vi "Main.vi"() -> ()   [LabVIEW 2020, in "Main.lvclass"]
uses:
  Main/Main.lvclass
  Support/Log Indicator/Log Indicator.lvclass
  C:/Program Files (x86)/National Instruments/LabVIEW 2020/vi.lib/Asteme/Triarc Framework/Logging/Logging.lvclass
  Main/Main.lvclass/Main.ctl
  Support/Log Indicator/Log Indicator.lvclass/Log Indicator.ctl
  <vilib>/Asteme/Triarc Framework/Process/Process.lvclass/Process.ctl
  <vilib>/Asteme/Triarc Framework/Process/Private/SubVIs/Wait for finish.vi
  <vilib>/Asteme/Triarc Framework/Process/Protected/Messaging/Enqueue Message.vi
  <vilib>/Asteme/Triarc Framework/Process/Private/SubVIs/Set Lifecycle State.vi
  <vilib>/Asteme/Triarc Framework/Process/Public/Lifecycle/Get Lifecycle State.vi
  <vilib>/Utility/error.llb/Clear Errors.vi
  Processes/Coffee Shop/Coffee Shop.lvclass
  C:/Program Files (x86)/National Instruments/LabVIEW 2020/vi.lib/Asteme/Triarc Framework/Process/Process.lvclass
  C:/Program Files (x86)/National Instruments/LabVIEW 2020/vi.lib/Asteme/Triarc Framework/Application/Application.lvclass
  <vilib>/Utility/error.llb/Error Cluster From Error Code.vi
  <vilib>/Asteme/Triarc Framework/Application/Application.lvclass
  <vilib>/Asteme/Triarc Framework/Process/Process.lvclass
panel:
  in  "Has Phone?":bool=TRUE
  out "System Log":string
  in  "Remove Customer":bool
  in  "Stop Button":bool
  in  "Remove Barista":bool
  in  "Show Barista Info":bool
  in  "Add Barista":bool
  in  "Baristas":i32(listbox)=-1
  in  "Remove Cashier":bool
  in  "Show Cashier Info":bool
  in  "Add Cashier":bool
  in  "Cashiers":i32(listbox)=-1
  in  "Show Customer Info":bool
  in  "Add Customer":bool
  in  "Customers":i32(listbox)=-1
  # "Click + to add a customer actor to the system.\nClick Place Order to choose items for the customer to order.\nCustomer will wait until all items ordered are ready, then exit."
  # "Cashiers process orders into individual drink jobs and forwards those jobs to baristas.\nClick + to add a cashier actor to the system.\nClick - to remove a cashier from the system."
  # "Baristas process drink jobs and notify customers of completed drinks.\nAdd more baristas to the system by clicking +.  Pending jobs will be assigned to the next available barista.\nClick - to remove a barista from the system."
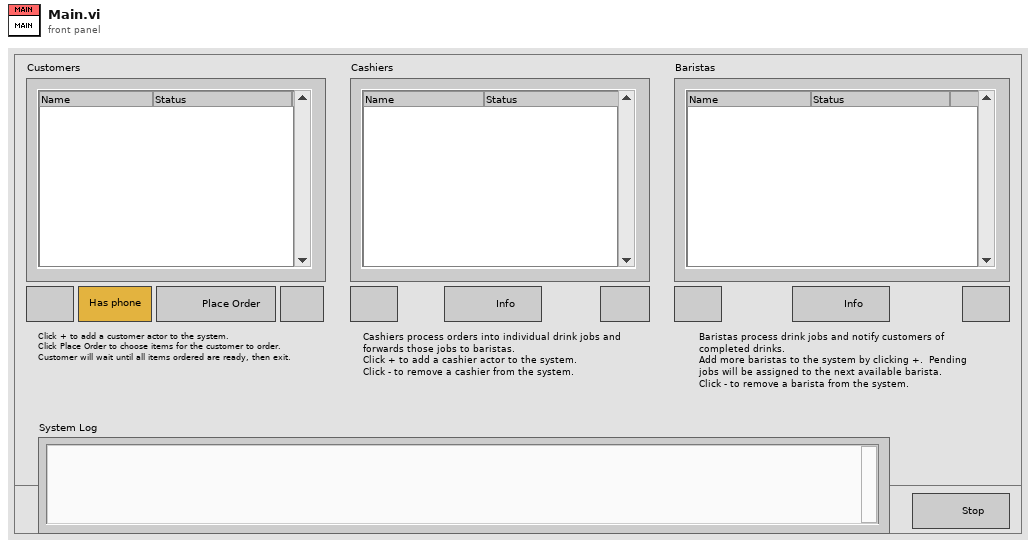
[diagram p1: front panel]
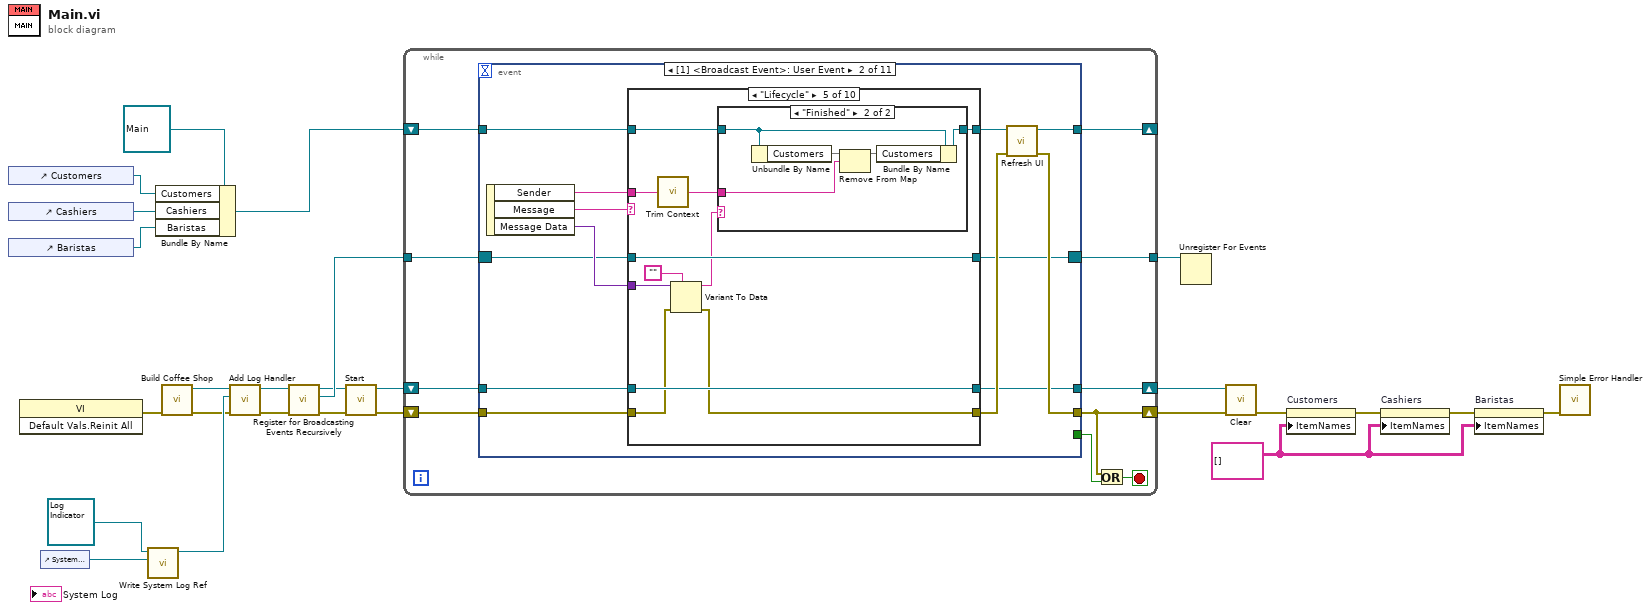
[diagram p0: block diagram]
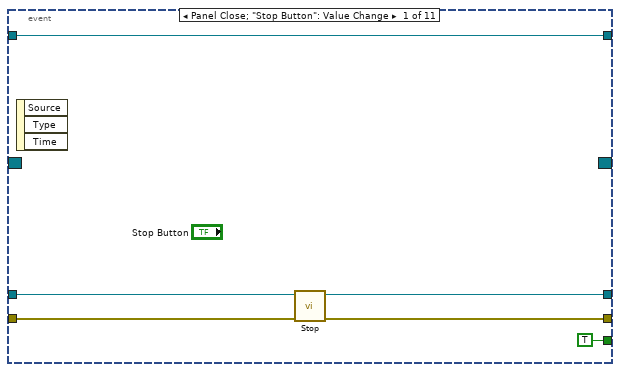
[diagram p2: hidden frame]
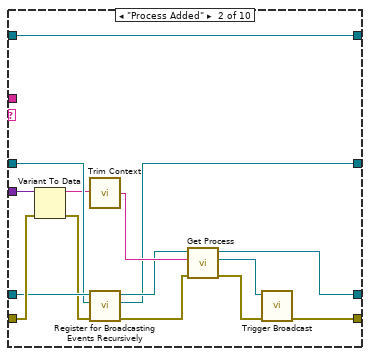
[diagram p4: hidden frame]
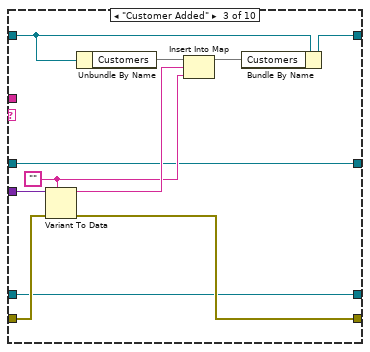
[diagram p5: hidden frame]
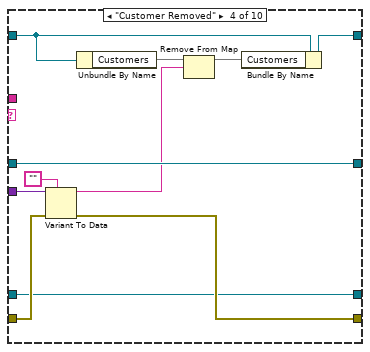
[diagram p6: hidden frame]
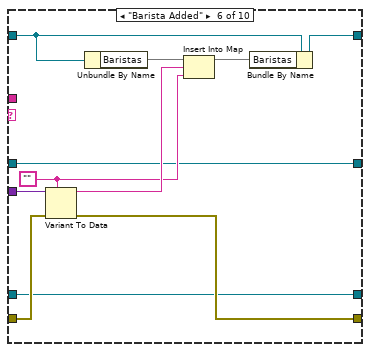
[diagram p8: hidden frame]
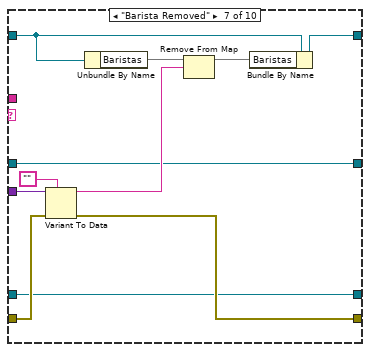
[diagram p9: hidden frame]
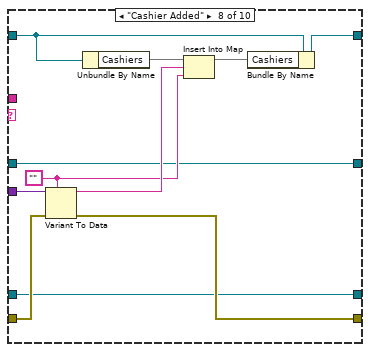
[diagram p10: hidden frame]
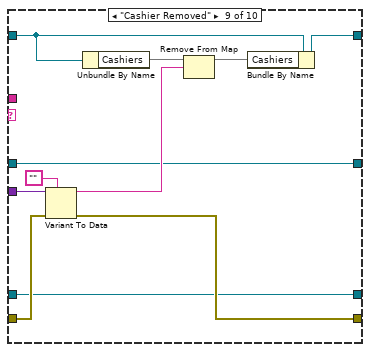
[diagram p11: hidden frame]
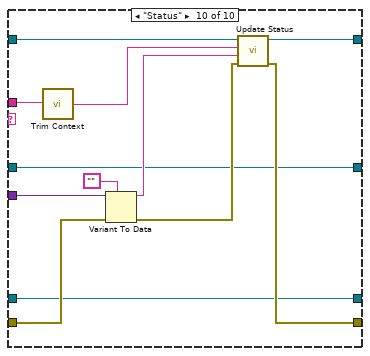
[diagram p12: hidden frame]
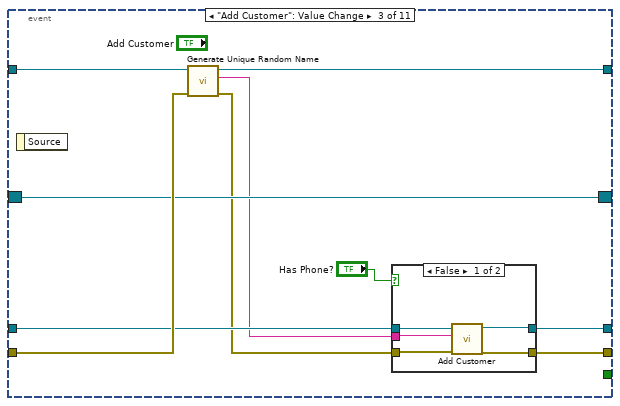
[diagram p13: hidden frame]
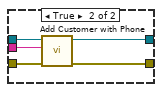
[diagram p14: hidden frame]
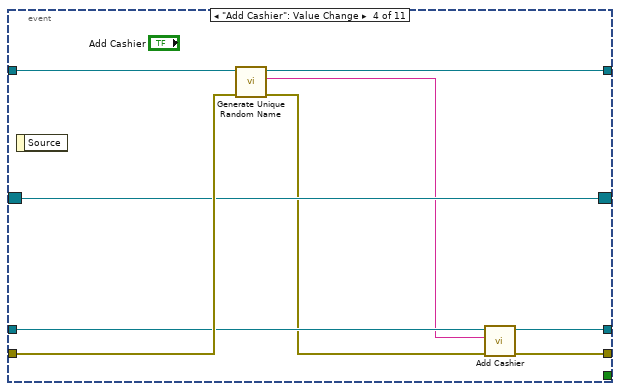
[diagram p15: hidden frame]
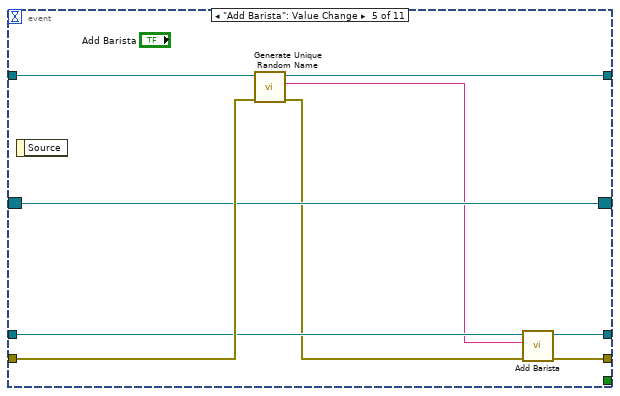
[diagram p16: hidden frame]
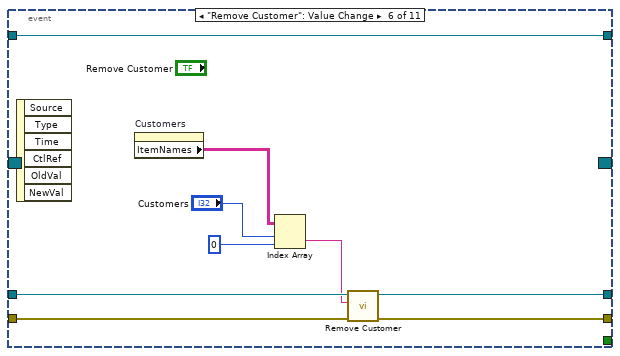
[diagram p17: hidden frame]
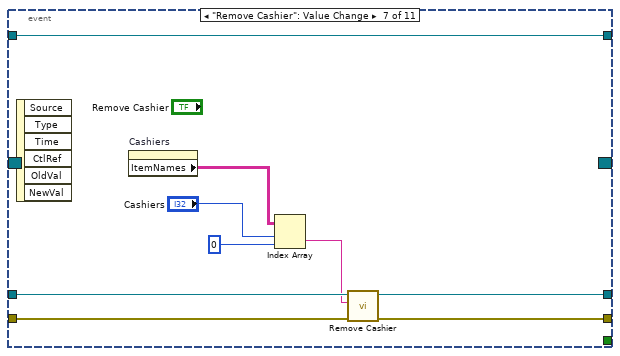
[diagram p18: hidden frame]
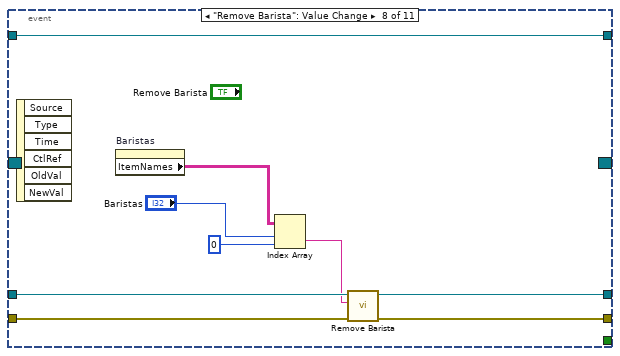
[diagram p19: hidden frame]
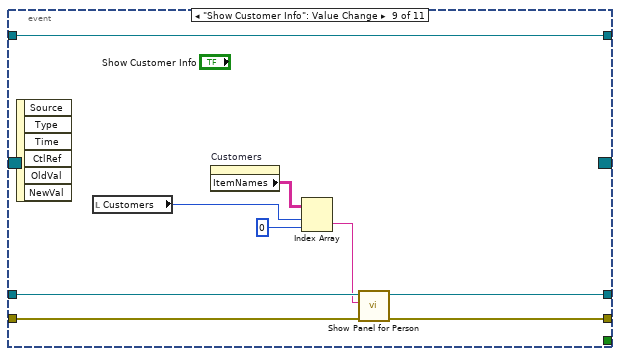
[diagram p20: hidden frame]
diagram:
  w8 = string[][] [] ("Item Names")
  n1 = control-ref of="Customers"() -> (w20:refnum<vi>)
  n2 = control-ref of="Cashiers"() -> (w19:refnum<vi>)
  n3 = control-ref of="Baristas"() -> (w18:refnum<vi>)
  n4 = invoke on="Invoke Node" class="VI" method="Default Vals.Reinit All"() -> (error out=w23:errorcluster)  [unwired: 3 in, 2 out]
  n5 = control-ref of="System Log"() -> (w14:refnum<vi>)
  n6 = call "Write System Log Ref.vi"("System Log"=w14, "Log Indicator in"=refnum<class "Log Indicator.lvclass"> refnum ("Log Indicator.lvclass")) -> ("Log Indicator out"=w12:refnum<class "Log Indicator.lvclass">)  [unwired: 8 in, 1 out]
  n7 = Bundle By Name(cluster=refnum<class "Main.lvclass"> refnum ("Main.lvclass"), "Customers"=w20, "Cashiers"=w19, "Baristas"=w18) -> (w21:refnum<class "Main.lvclass">)
  n8 = call "Build Coffee Shop.vi"("error in (no error)"=w23) -> ("error out"=w10:errorcluster, "Coffee Shop Out"=w11:refnum<class "Coffee Shop.lvclass">)  [unwired: 9 in]
  n9 = call <vilib>:"Add Log Handler.vi"("error in (no error)"=w10, "Log Handler"=w12, "Process In"=w11) -> ("error out"=w13:errorcluster, "Process Out"=w9:refnum<class "Coffee Shop.lvclass">)  [unwired: 7 in]
  n10 = call <vilib>:"Register for Broadcasting Events Recursively.vi"("error in (no error)"=w13, "Application In"=w9) -> ("error out"=w17:errorcluster, "Event Registration Refnum Out"=w16:refnum<event-registration>, "Application Out"=w3:refnum<class "Coffee Shop.lvclass">)  [unwired: 7 in]
  n11 = call <vilib>:"Start.vi"("error in (no error)"=w17, "Process In"=w3) -> ("error out"=w4:errorcluster, "Process Out"=w2:refnum<class "Coffee Shop.lvclass">)  [unwired: 8 in]
  n12 = while {
    shift-right: [w35] -> w25
    shift-left: w4 -> [w36]
    shift-right: [w31] -> w24
    shift-left: w2 -> [w32]
    tunnel: w16 -> [w30]
    tunnel: [w29] -> w26
    shift-right: [w27] -> _
    shift-left: w21 -> [w28]
    stop <- w34 stop-if-true
    n13 = event shown="[1] <Broadcast Event>: User Event" {
      selector: w30 -> [_ w44 w177 w196 w205 _ _ _ _ _ _]
      dyn-events: [_ w43 w177 w196 w205 _ _ _ _ _ _] -> w29
      timeout: _ -> [_ _ _ _ _ _ _ _ _ _ _]
      tunnel: [w40 w50 w175 w194 w203 w215 w224 w233 w238 w247 w256] -> w35
      tunnel: w36 -> [w42 w52 w179 w198 w207 w214 w223 w232 w243 w252 w261]
      tunnel: [TRUE _ _ _ _ _ _ _ _ _ _] -> w33
      tunnel: w32 -> [w39 w45 w178 w197 w206 w212 w221 w230 w237 w246 w255]
      tunnel: [w38 w46 w176 w195 w204 w213 w222 w231 w236 w245 w254] -> w31
      tunnel: w28 -> [w37 w51 w172 w192 w201 w216 w225 w234 w242 w251 w260]
      tunnel: [w37 w48 w171 w191 w200 w216 w225 w234 w242 w251 w260] -> w27
      event Panel Close; "Stop Button": Value Change {
        n14 = event-data() -> ()  [unwired: 1 in, 3 out]
        n15 = call <vilib>:"Stop.vi"("error in (no error)"=w42, "Process In"=w39) -> ("error out"=w40:errorcluster, "Process Out"=w38:refnum<class "Coffee Shop.lvclass">)  [unwired: 7 in, 1 out]
      }
      event User Event {
        n16 = event-data() -> ("Sender"=w47:string, "Message"=w55:string, "Message Data"=w54:variant)  [unwired: 1 in]
        n17 = case shown="\"Lifecycle\"" w55 {
          tunnel: w54 -> [_ w61 w85 w96 w103 w124 w135 w146 w157 w162]
          tunnel: w52 -> [w59 w68 w84 w95 w100 w123 w134 w145 w156 w165]
          tunnel: [w59 w71 w83 w94 w101 w122 w133 w144 w155 w166] -> w53
          tunnel: w51 -> [w58 w74 w82 w93 w107 w121 w132 w143 w154 w167]
          tunnel: [w58 w74 w80 w92 w106 w119 w130 w141 w152 w168] -> w49
          tunnel: w47 -> [_ _ _ _ w97 _ _ _ _ w169]
          tunnel: [w57 w70 w76 w90 w105 w115 w126 w137 w148 w159] -> w46
          tunnel: w45 -> [w57 w65 w76 w90 w105 w115 w126 w137 w148 w159]
          tunnel: w44 -> [w56 w64 w75 w89 w104 w114 w125 w136 w147 w158]
          tunnel: [w56 w63 w75 w89 w104 w114 w125 w136 w147 w158] -> w43
          frame Default {
          }
          frame "Process Added" {
            n18 = Variant To Data(error in=w68, Variant=w61) -> (data=w60:string, error out=w62:errorcluster)  [unwired: 1 in]
            n19 = call "Trim Context.vi"("Qualified Name"=w60) -> ("Name"=w72:string)
            n20 = call <vilib>:"Register for Broadcasting Events Recursively.vi"("error in (no error)"=w62, "Event Registration Refnum In"=w64, "Application In"=w65) -> ("error out"=w67:errorcluster, "Event Registration Refnum Out"=w63:refnum<event-registration>, "Application Out"=w66:refnum<class "Coffee Shop.lvclass">)  [unwired: 6 in]
            n21 = call <vilib>:"Get Process.vi"("error in (no error)"=w67, "Process Name"=w72, "Rig In"=w66) -> ("error out"=w73:errorcluster, "App Process"=w69:refnum<class "Process.lvclass">, "Rig Out"=w70:refnum<class "Coffee Shop.lvclass">)  [unwired: 6 in]
            n22 = call <vilib>:"Trigger Broadcast.vi"("error in (no error)"=w73, "Process in"=w69) -> ("error out"=w71:errorcluster)  [unwired: 8 in, 1 out]
          }
          frame "Customer Added" {
            w77 = ""
            n23 = Variant To Data(error in=w84, type=w77, Variant=w85) -> (data=w78:string, error out=w83:errorcluster)
            n24 = Unbundle By Name(w82) -> ("Customers"=w81:map{string, string})
            n25 = Insert Into Map(map in=w81, key=w78, value=w77) -> (map out=w79:map{string, string})  [unwired: 2 out]
            n26 = Bundle By Name(cluster=w82, "Customers"=w79) -> (w80:refnum<class "Main.lvclass">)
          }
          frame "Customer Removed" {
            n27 = Variant To Data(error in=w95, type="", Variant=w96) -> (data=w88:string, error out=w94:errorcluster)
            n28 = Unbundle By Name(w93) -> ("Customers"=w87:map{string, string})
            n29 = Remove From Map(10:w88, 11:w87) -> (3:w86:map{string, string})  [unwired: 2 out]
            n30 = Bundle By Name(cluster=w93, "Customers"=w86) -> (w92:refnum<class "Main.lvclass">)
          }
          frame "Lifecycle" {
            n31 = call "Trim Context.vi"("Qualified Name"=w97) -> ("Name"=w98:string)
            n32 = Variant To Data(error in=w100, type="", Variant=w103) -> (data=w99:string, error out=w101:errorcluster)
            n33 = case shown="\"Finished\"" w99 {
              tunnel: w107 -> [w108 w113]
              tunnel: [w108 w112] -> w106
              tunnel: w98 -> [_ w109]
              frame Default {
              }
              frame "Finished" {
                n34 = Unbundle By Name(w113) -> ("Customers"=w111:map{string, string})
                n35 = Remove From Map(10:w109, 11:w111) -> (3:w110:map{string, string})  [unwired: 2 out]
                n36 = Bundle By Name(cluster=w113, "Customers"=w110) -> (w112:refnum<class "Main.lvclass">)
              }
            }
          }
          frame "Barista Added" {
            w116 = ""
            n37 = Variant To Data(error in=w123, type=w116, Variant=w124) -> (data=w117:string, error out=w122:errorcluster)
            n38 = Unbundle By Name(w121) -> ("Baristas"=w120:map{string, string})
            n39 = Insert Into Map(map in=w120, key=w117, value=w116) -> (map out=w118:map{string, string})  [unwired: 2 out]
            n40 = Bundle By Name(cluster=w121, "Baristas"=w118) -> (w119:refnum<class "Main.lvclass">)
          }
          frame "Barista Removed" {
            n41 = Variant To Data(error in=w134, type="", Variant=w135) -> (data=w128:string, error out=w133:errorcluster)
            n42 = Unbundle By Name(w132) -> ("Baristas"=w131:map{string, string})
            n43 = Remove From Map(10:w128, 11:w131) -> (3:w129:map{string, string})  [unwired: 2 out]
            n44 = Bundle By Name(cluster=w132, "Baristas"=w129) -> (w130:refnum<class "Main.lvclass">)
          }
          frame "Cashier Added" {
            w138 = ""
            n45 = Variant To Data(error in=w145, type=w138, Variant=w146) -> (data=w139:string, error out=w144:errorcluster)
            n46 = Unbundle By Name(w143) -> ("Cashiers"=w142:map{string, string})
            n47 = Insert Into Map(map in=w142, key=w139, value=w138) -> (map out=w140:map{string, string})  [unwired: 2 out]
            n48 = Bundle By Name(cluster=w143, "Cashiers"=w140) -> (w141:refnum<class "Main.lvclass">)
          }
          frame "Cashier Removed" {
            n49 = Variant To Data(error in=w156, type="", Variant=w157) -> (data=w150:string, error out=w155:errorcluster)
            n50 = Unbundle By Name(w154) -> ("Cashiers"=w153:map{string, string})
            n51 = Remove From Map(10:w150, 11:w153) -> (3:w151:map{string, string})  [unwired: 2 out]
            n52 = Bundle By Name(cluster=w154, "Cashiers"=w151) -> (w152:refnum<class "Main.lvclass">)
          }
          frame "Status" {
            n53 = call "Trim Context.vi"("Qualified Name"=w169) -> ("Name"=w164:string)
            n54 = Variant To Data(error in=w165, type="", Variant=w162) -> (data=w160:string, error out=w163:errorcluster)
            n55 = call "Update Status.vi"("error in (no error)"=w163, "Status"=w160, "Name"=w164, "Main In"=w167) -> ("error out"=w166:errorcluster, "Main Out"=w168:refnum<class "Main.lvclass">)  [unwired: 6 in]
          }
        }
        n56 = call "Refresh UI.vi"("error in (no error)"=w53, "Main in"=w49) -> ("error out"=w50:errorcluster, "Main out"=w48:refnum<class "Main.lvclass">)  [unwired: 8 in]
      }
      event "Add Customer": Value Change {
        n57 = event-data() -> ()  [unwired: 1 in, 1 out]
        n58 = call "Generate Unique Random Name.vi"("error in (no error)"=w179, "Main in"=w172) -> ("error out"=w173:errorcluster, "Name"=w170:string, "Main out"=w171:refnum<class "Main.lvclass">)  [unwired: 7 in]
        n59 = case shown="False" "Has Phone?" {
          tunnel: w173 -> [w183 w189]
          tunnel: w178 -> [w184 w188]
          tunnel: w170 -> [w180 w187]
          tunnel: [w182 w186] -> w176
          tunnel: [w181 w185] -> w175
          frame False {
            n60 = call "Add Customer.vi"("error in (no error)"=w183, "Name"=w180, "Coffee Shop in"=w184) -> ("error out"=w181:errorcluster, "Coffee Shop out"=w182:refnum<class "Coffee Shop.lvclass">)  [unwired: 7 in]
          }
          frame True {
            n61 = call "Add Customer with Phone.vi"("error in (no error)"=w189, "Name"=w187, "Coffee Shop in"=w188) -> ("error out"=w185:errorcluster, "Coffee Shop out"=w186:refnum<class "Coffee Shop.lvclass">)  [unwired: 7 in]
          }
        }
      }
      event "Add Cashier": Value Change {
        n62 = event-data() -> ()  [unwired: 1 in, 1 out]
        n63 = call "Generate Unique Random Name.vi"("error in (no error)"=w198, "Main in"=w192) -> ("error out"=w193:errorcluster, "Name"=w190:string, "Main out"=w191:refnum<class "Main.lvclass">)  [unwired: 7 in]
        n64 = call "Add Cashier.vi"("error in (no error)"=w193, "Name"=w190, "Coffee Shop in"=w197) -> ("error out"=w194:errorcluster, "Coffee Shop out"=w195:refnum<class "Coffee Shop.lvclass">)  [unwired: 7 in]
      }
      event "Add Barista": Value Change {
        n65 = event-data() -> ()  [unwired: 1 in, 1 out]
        n66 = call "Generate Unique Random Name.vi"("error in (no error)"=w207, "Main in"=w201) -> ("error out"=w202:errorcluster, "Name"=w199:string, "Main out"=w200:refnum<class "Main.lvclass">)  [unwired: 7 in]
        n67 = call "Add Barista.vi"("error in (no error)"=w202, "Name"=w199, "Coffee Shop in"=w206) -> ("error out"=w203:errorcluster, "Coffee Shop out"=w204:refnum<class "Coffee Shop.lvclass">)  [unwired: 7 in]
      }
      event "Remove Customer": Value Change {
        n68 = event-data() -> ()  [unwired: 1 in, 6 out]
        n69 = property on="Customers" class="MCListbox (strict)"() -> ("ItemNames"=w211:string[][])  [unwired: 2 in, 2 out]
        n70 = Index Array(array=w211, index (row)="Customers", index (col)=0 ("disabled index (col)")) -> (element=w208:string)
        n71 = call "Remove Customer.vi"("error in (no error)"=w214, "Name"=w208, "Coffee Shop In"=w212) -> ("error out"=w215:errorcluster, "Coffee Shop Out"=w213:refnum<class "Coffee Shop.lvclass">)  [unwired: 7 in]
      }
      event "Remove Cashier": Value Change {
        n72 = event-data() -> ()  [unwired: 1 in, 6 out]
        n73 = property on="Cashiers" class="MCListbox (strict)"() -> ("ItemNames"=w217:string[][])  [unwired: 2 in, 2 out]
        n74 = Index Array(array=w217, index (row)="Cashiers", index (col)=0 ("disabled index (col)")) -> (element=w219:string)
        n75 = call "Remove Cashier.vi"("error in (no error)"=w223, "Name"=w219, "Coffee Shop In"=w221) -> ("error out"=w224:errorcluster, "Coffee Shop Out"=w222:refnum<class "Coffee Shop.lvclass">)  [unwired: 7 in]
      }
      event "Remove Barista": Value Change {
        n76 = event-data() -> ()  [unwired: 1 in, 6 out]
        n77 = property on="Baristas" class="MCListbox (strict)"() -> ("ItemNames"=w226:string[][])  [unwired: 2 in, 2 out]
        n78 = Index Array(array=w226, index (row)="Baristas", index (col)=0 ("disabled index (col)")) -> (element=w228:string)
        n79 = call "Remove Barista.vi"("error in (no error)"=w232, "Name"=w228, "Coffee Shop In"=w230) -> ("error out"=w233:errorcluster, "Coffee Shop Out"=w231:refnum<class "Coffee Shop.lvclass">)  [unwired: 7 in]
      }
      event "Show Customer Info": Value Change {
        n80 = event-data() -> ()  [unwired: 1 in, 6 out]
        n81 = local read "Customers"() -> (w240:i32)
        n82 = property on="Customers" class="MCListbox (strict)"() -> ("ItemNames"=w241:string[][])  [unwired: 2 in, 2 out]
        n83 = Index Array(array=w241, index (row)=w240, index (col)=0 ("disabled index (col)")) -> (element=w235:string)
        n84 = call "Show Panel for Person.vi"("error in (no error)"=w243, "Name"=w235, "Coffee Shop In"=w237) -> ("error out"=w238:errorcluster, "Coffee Shop Out"=w236:refnum<class "Coffee Shop.lvclass">)  [unwired: 7 in]
      }
      event "Show Cashier Info": Value Change {
        n85 = event-data() -> ()  [unwired: 1 in, 6 out]
        n86 = local read "Cashiers"() -> (w249:i32)
        n87 = property on="Cashiers" class="MCListbox (strict)"() -> ("ItemNames"=w250:string[][])  [unwired: 2 in, 2 out]
        n88 = Index Array(array=w250, index (row)=w249, index (col)=0 ("disabled index (col)")) -> (element=w244:string)
        n89 = call "Show Panel for Person.vi"("error in (no error)"=w252, "Name"=w244, "Coffee Shop In"=w246) -> ("error out"=w247:errorcluster, "Coffee Shop Out"=w245:refnum<class "Coffee Shop.lvclass">)  [unwired: 7 in]
      }
      event "Show Barista Info": Value Change {
        n90 = event-data() -> ()  [unwired: 1 in, 6 out]
        n91 = local read "Baristas"() -> (w258:i32)
        n92 = property on="Baristas" class="MCListbox (strict)"() -> ("ItemNames"=w259:string[][])  [unwired: 2 in, 2 out]
        n93 = Index Array(array=w259, index (row)=w258, index (col)=0 ("disabled index (col)")) -> (element=w253:string)
        n94 = call "Show Panel for Person.vi"("error in (no error)"=w261, "Name"=w253, "Coffee Shop In"=w255) -> ("error out"=w256:errorcluster, "Coffee Shop Out"=w254:refnum<class "Coffee Shop.lvclass">)  [unwired: 7 in]
      }
    }
    n95 = Or(x=w35, y=w33) -> (x .or. y?=w34:bool)
  }
  n96 = Unregister For Events(event registration refnum=w26) -> ()  [unwired: 1 in, 1 out]
  n97 = call-dynamic "Clear.vi"("error in (no error)"=w25, "Application In"=w24) -> ("error out"=w5:errorcluster)  [unwired: 9 in]
  n98 = property on="Customers" class="MCListbox (strict)"(error in=w5, "ItemNames"=w8) -> (error out=w6:errorcluster)  [unwired: 1 in, 1 out]
  n99 = property on="Cashiers" class="MCListbox (strict)"(error in=w6, "ItemNames"=w8) -> (error out=w7:errorcluster)  [unwired: 1 in, 1 out]
  n100 = property on="Baristas" class="MCListbox (strict)"(error in=w7, "ItemNames"=w8) -> (error out=w1:errorcluster)  [unwired: 1 in, 1 out]
  n101 = call <vilib>:"Simple Error Handler.vi"("error in (no error)"=w1) -> ()  [unwired: 4 in, 5 out]
